vi "Load Classes from Disk.vi"(8 "error in (no error)":errorcluster, 10 "class paths":path[](array[path]), 11 "Transceiver Loader in":refnum<class "Transceiver Loader.lvclass">) -> (0 "error out":errorcluster, 2 "Transceivers":refnum<class "Transceiver.lvclass">[](array[class]), 3 "Transceiver Loader out":refnum<class "Transceiver Loader.lvclass">)   [LabVIEW 2017, in "Data Sharing Framework Core.lvlib" / "Data Sharing Framework Engine.lvlib" / "Transceiver Loader.lvclass"]
uses:
  Transceiver Loader.lvclass
  Transceiver/Transceiver.lvclass
  Configuration Classes/Transceiver Configuration/Transceiver Configuration.lvclass
panel:
  out "Transceiver Configurations":refnum<class "Transceiver Configuration.lvclass">[](array[class])
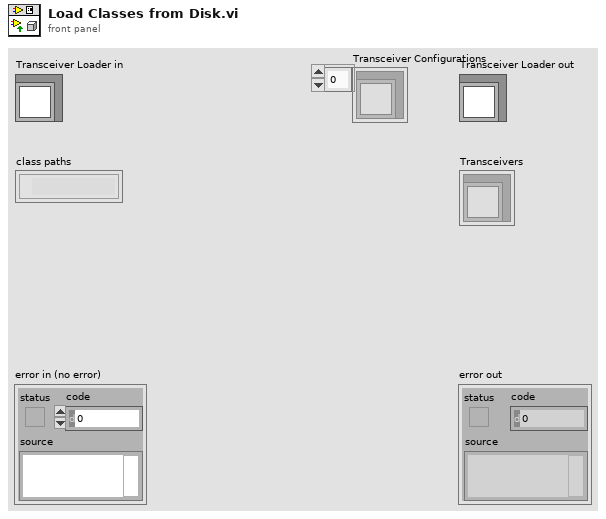
[diagram p1: front panel]
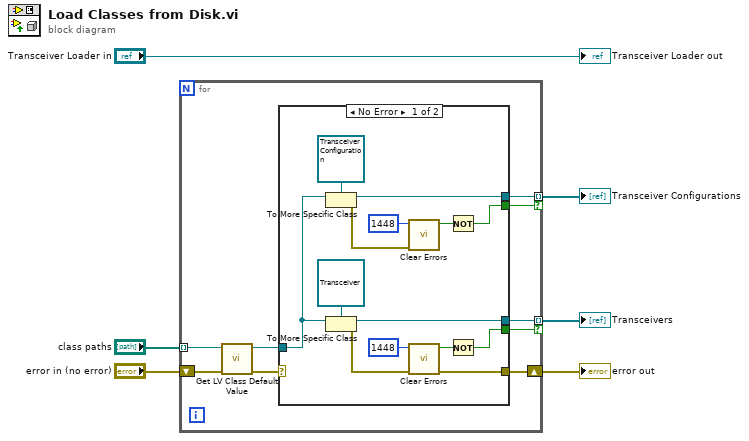
[diagram p0: block diagram]
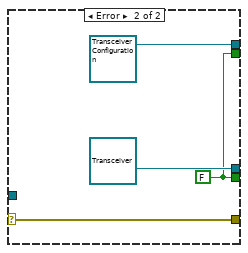
[diagram p2: hidden frame]
diagram:
  n1 = for {
    tunnel: "class paths" -> [w15] mode=indexing
    shift-right: [w9] -> w5
    shift-left: "error in (no error)" -> [w14]
    tunnel: [w12] -> w2 mode=indexing if=w10
    tunnel: [w8] -> w1 mode=indexing if=w7
    n2 = call <vilib>:"Get LV Class Default Value.vi"("error in (no error)"=w14, "class path"=w15) -> ("error out"=w11:errorcluster, "object"=w13:refnum<class>)  [unwired: 8 in]
    n3 = case shown="No Error" w11 {
      selector: w11 -> [_ w32]
      tunnel: w13 -> [w23 _]
      tunnel: [w24 refnum<class "Transceiver.lvclass"> refnum ("DSF.Engine.lvlib:Transceiver")] -> w12
      tunnel: [w18 w30] -> w10
      tunnel: [w26 w32] -> w9
      tunnel: [w19 refnum<class "Transceiver Configuration.lvclass"> refnum ("DSF.Engine.lvlib:DSF.Shared.Configuration.Transceiver.lvclass")] -> w8
      tunnel: [w17 w30] -> w7
      frame No Error {
        n4 = To More Specific Class(target class=refnum<class "Transceiver Configuration.lvclass"> refnum ("DSF.Engine.lvlib:DSF.Shared.Configuration.Transceiver.lvclass"), reference=w23) -> (specific class reference=w19:refnum<class "Transceiver Configuration.lvclass">, error out=w20:errorcluster)  [unwired: 1 in]
        n5 = To More Specific Class(target class=refnum<class "Transceiver.lvclass"> refnum ("DSF.Engine.lvlib:Transceiver"), reference=w23) -> (specific class reference=w24:refnum<class "Transceiver.lvclass">, error out=w28:errorcluster)  [unwired: 1 in]
        n6 = call <vilib>:"Clear Errors.vi"("error in (no error)"=w20, "specific error code to clear (0: all)"=1448) -> ("specific error cleared?"=w16:bool)  [unwired: 4 in, 1 out]
        n7 = call <vilib>:"Clear Errors.vi"("error in (no error)"=w28, "specific error code to clear (0: all)"=1448) -> ("error out"=w26:errorcluster, "specific error cleared?"=w27:bool)  [unwired: 4 in]
        n8 = Not(x=w16) -> (.not. x?=w17:bool)
        n9 = Not(x=w27) -> (.not. x?=w18:bool)
      }
      frame Error {
        w30 = FALSE
      }
    }
  }
  "error out" <- w5
  "Transceivers" <- w2
  "Transceiver Configurations" <- w1
  "Transceiver Loader out" <- "Transceiver Loader in"
